vi "Motor with Encoder.vi"() -> ()   [LabVIEW 2016]
doc: "This example shows how to move a motor connected to an encoder and a wheel, and then read information about the system from an encoder.\n\nThis is an example of how to use feedback (from the encoder) to create an open loop system. If some control method was used, for example using PID, a closed loop system could be created.\n\nThis example expects a USB cable connected from your development PC to the Type B USB Jack (next to the power input) on the roboRIO.\n\nThis example requires the Driver Station to be running with Teleoperated Enabled."
uses:
  <vilib>/Rock Robotics/SystemInterfaces/DIO/FPGA_DIOChannel.ctl
  <vilib>/Rock Robotics/WPI/Encoder/WPI_EncoderType.ctl
  <vilib>/Rock Robotics/SystemInterfaces/DIO/FPGA_DIOPWMChannel.ctl
  <vilib>/Rock Robotics/WPI/Counter/WPI_CounterDigitalInputToDigitalSource.vi
  <vilib>/Rock Robotics/WPI/MotorControl/WPI_MotorControlOpen Talon.vi
panel:
  out "Current angle (deg)":dbl(knob) scale=0.0..360.0
  out "Distance (in)":dbl
  out "Revolutions":dbl
  in  "Wheel diameter (in)":dbl=6.0
  in  "Motor Speed (-1 to 1)":dbl(slide) scale=-1.0..1.0
  in  "Motor PWM Channel":T1
  in  "Number Samples to Average":u8=1 min=1 max=128
  in  "Invert Direction":bool
  in  "Decoding Type":T2=enum."4x"
  in  "DistancePerCount (deg)":dbl=0.288
  in  "Encoder B Channel":T3=enum."DIO 1"
  in  "Encoder A Channel":T3
  out "Encoder Rate (deg/sec)":dbl
  in  "Minimum Rate":dbl=20.0
  in  "Stop":bool
  in  "Reset Encoder?":bool
  out "Encoder Alarm Status":string
  out "Encoder Direction":string
  # "Set these inputs before running."
  # "These can be set while running."
  # "Output information."
  # "This example requires the Driver Station to be running with Teleoperated Enabled."
  # "PWM cable"
  # "This shows wiring for a Talon speed controller.  The wiring is similar for Victor and Jaguar controllers.  If you change the controller type, you must also select the appropriate instance of the Motor Open VI on the diagram."
  # "Power\nTerminals"
  # "Motor\nTerminals"
  # "+"
  # "+"
  # "M"
  # "B"
  # "Encoder\nB (white wire)---------\nGnd (black wire)------\n+5V (red wire)---------\nA (white wire)---------"
  # "roboRIO\nDIO-1  S\nDIO-0 \nDIO-0  V\nDIO-0  S"
  # "Encoder"
  # "Index"
  # "Gnd"
  # "+5V"
  # "B"
  # "A"
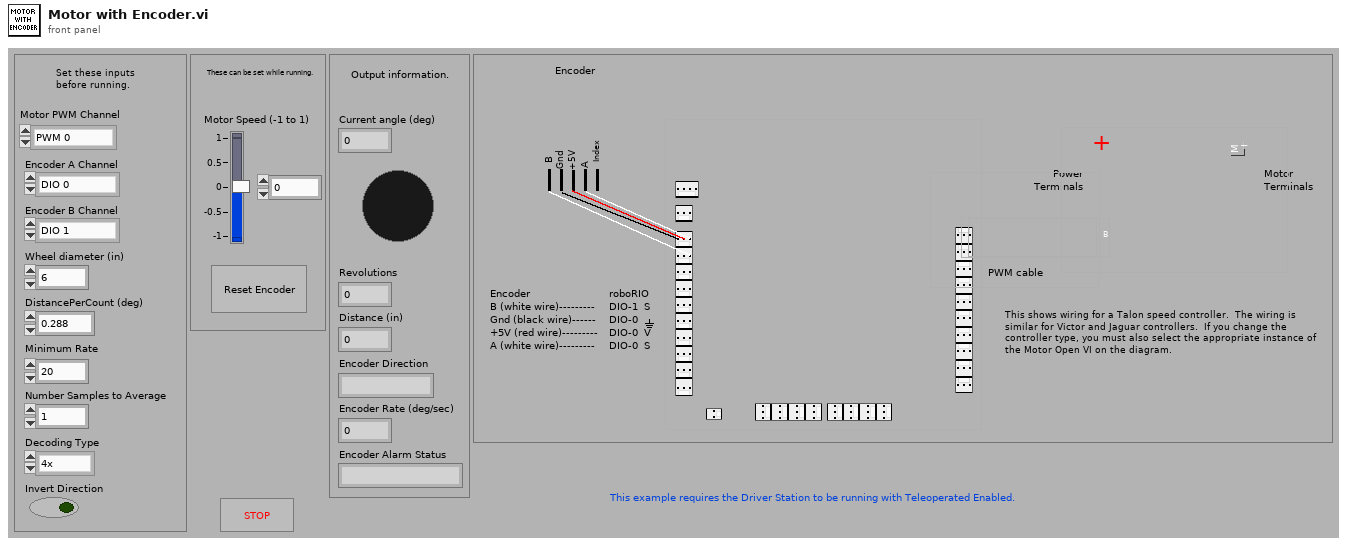
[diagram p1: front panel]
types:
  T1 = typedef "FPGA_DIOPWMChannel.ctl" = enum8{"PWM 0", "PWM 1", "PWM 2", "PWM 3", "PWM 4", "PWM 5", "PWM 6", "PWM 7", "PWM 8", "PWM 9", "PWM MXP 0", "PWM MXP 1", "PWM MXP 2", "PWM MXP 3", "PWM MXP 4", "PWM MXP 5", "PWM MXP 6", "PWM MXP 7", "PWM MXP 8", "PWM MXP 9", "Invalid"}
  T2 = typedef "WPI_EncoderType.ctl" = enum16{"1x", "2x", "4x"}
  T3 = typedef "FPGA_DIOChannel.ctl" = enum8{"DIO 0", "DIO 1", "DIO 2", "DIO 3", "DIO 4", "DIO 5", "DIO 6", "DIO 7", "DIO 8", "DIO 9", "DIO MXP 0", "DIO MXP 1", "DIO MXP 2", "DIO MXP 3", "DIO MXP 4", "DIO MXP 5", "DIO MXP 6", "DIO MXP 7", "DIO MXP 8", "DIO MXP 9", "DIO MXP 10", "DIO MXP 11", "DIO MXP 12", "DIO MXP 13", "DIO MXP 14", "DIO MXP 15", "SPI Port CS1", "SPI Port CS2", "SPI Port CS3", "SPI Port MISO", "SPI Port MOSI", "Invalid"}
  T4 = typedef "WPI_MotorControlDeviceRef.ctl" = cluster{"DeviceStatus":errorcluster, "Type":T5, "PWM":cluster{"PWM Channel":T1, "DeadBand":T6}, "CAN":cluster{"Device Number":u8, "SetOutput VI Ref":variant, "GetOutput VI Ref":variant, "Enable VI Ref":variant, "Disable VI Ref":variant, "Data":variant}, "Invert":bool}
  T5 = typedef "WPI_MotorControlType.ctl" = enum16{"PWM", "CAN"}
  T6 = typedef "WPI_PWMDeadband.ctl" = cluster{"Name":string, "maxPositivePwm":i32, "minPositivePwm":i32, "centerPwm":i32, "maxNegativePwm":i32, "minNegativePwm":i32, "angularRange":u16}
  T7 = typedef "WPI_DigitalInputDevRef.ctl" = cluster{"DevStatus":errorcluster, "DIO Channel":T3}
  T8 = typedef "FPGA_CounterEncoderSourceConvertionLVSourceType.ctl" = cluster{"DevStatus":errorcluster, "AnalogTriggerMode?":bool, "DigitalMode":cluster{"DIO Channel":T9}, "AnalogTriggerMode":cluster{"AnalogTriggerIndex":T10, "OutputType":T11}}
  T9 = typedef "FPGA_DIODigitalSourceChannel.ctl" = enum8{"DIO 0", "DIO 1", "DIO 2", "DIO 3", "DIO 4", "DIO 5", "DIO 6", "DIO 7", "DIO 8", "DIO 9", "DIO MXP 0", "DIO MXP 1", "DIO MXP 2", "DIO MXP 3", "DIO MXP 4", "DIO MXP 5", "DIO MXP 6", "DIO MXP 7", "DIO MXP 8", "DIO MXP 9", "DIO MXP 10", "DIO MXP 11", "DIO MXP 12", "DIO MXP 13", "DIO MXP 14", "DIO MXP 15", "Disabled"}
  T10 = typedef "FPGA_AnalogTriggerIndex.ctl" = enum8{"Trig 0", "Trig 1", "Trig 2", "Trig 3", "Trig 4", "Trig 5", "Trig 6", "Trig 7", "Invalid"}
  T11 = typedef "FPGA_AnalogTriggerOutType.ctl" = enum16{"InWindow", "TriggerState", "Rising", "Falling"}
  T12 = typedef "WPI_EncoderDevRef.ctl" = cluster{"DevStatus":errorcluster, "EncoderIndex":T13, "CounterIndex":T14, "DistancePerCount":dbl, "Decoding Type":T2}
  T13 = typedef "FPGA_EncoderIdx.ctl" = enum8{"Enc 0", "Enc 1", "Enc 2", "Enc 3", "Enc 4", "Enc 5", "Enc 6", "Enc 7", "Invalid"}
  T14 = typedef "FPGA_CounterCtrSystemIndex.ctl" = enum8{"Ctr 0", "Ctr 1", "Ctr 2", "Ctr 3", "Ctr 4", "Ctr 5", "Ctr 6", "Ctr 7", "Invalid"}
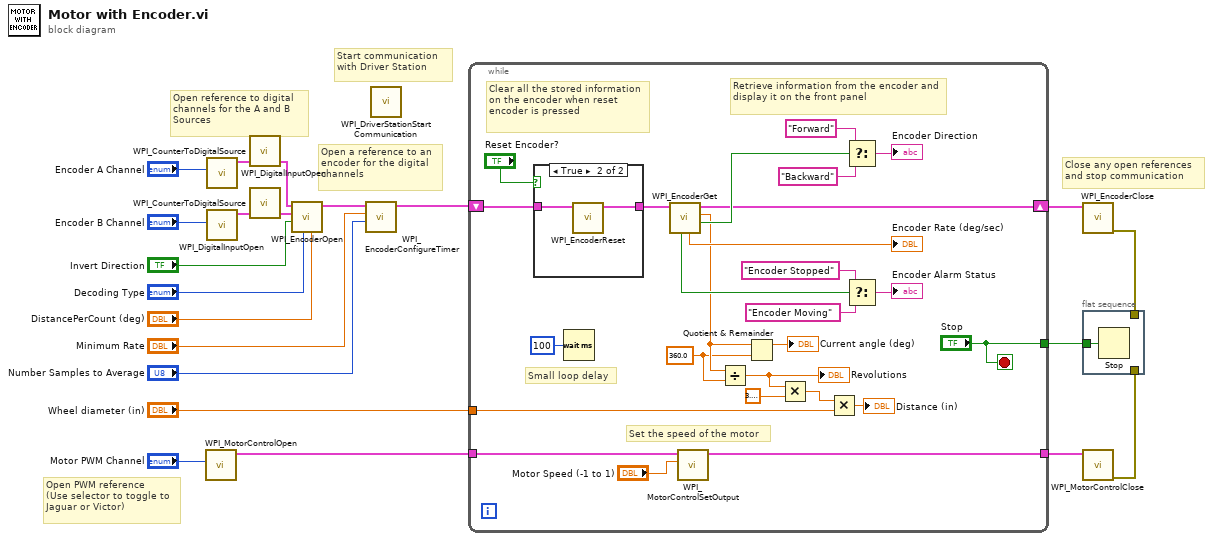
[diagram p0: block diagram]
diagram:
  # "Open PWM reference\n(Use selector to toggle to Jaguar or Victor)"
  # "Start communication with Driver Station"
  # "Close any open references\nand stop communication"
  # "Open a reference to an\nencoder for the digital \nchannels"
  # "Open reference to digital \nchannels for the A and B\nSources"
  n1 = call-poly <vilib>:"WPI_MotorControlOpen.vi"("PWM Channel"="Motor PWM Channel") -> ("MotorControlDeviceRef"=w5:T4)  [unwired: 3 in, 7 out]
  n2 = call <vilib>:"WPI_DigitalInputOpen.vi"("DIO Channel"="Encoder A Channel") -> ("DigitalInputDevRef"=w18:T7)  [unwired: 1 in, 9 out]
  n3 = call <vilib>:"WPI_DigitalInputOpen.vi"("DIO Channel"="Encoder B Channel") -> ("DigitalInputDevRef"=w19:T7)  [unwired: 1 in, 9 out]
  n4 = call-poly <vilib>:"WPI_CounterToDigitalSource.vi"("DigitalInputDevRef"=w18) -> ("Digital Source"=w17:T8)  [unwired: 6 out]
  n5 = call-poly <vilib>:"WPI_CounterToDigitalSource.vi"("DigitalInputDevRef"=w19) -> ("Digital Source"=w20:T8)  [unwired: 6 out]
  n6 = call <vilib>:"WPI_EncoderOpen.vi"("DistancePerCount"="DistancePerCount (deg)", "Decoding Type"="Decoding Type", "Invert Direction (False)"="Invert Direction", "BSource"=w20, "ASource"=w17) -> ("EncoderDevRef"=w10:T12)  [unwired: 3 in, 3 out]
  n7 = call <vilib>:"WPI_EncoderConfigureTimer.vi"("Number Samples to Average"="Number Samples to Average", "Minimum Rate"="Minimum Rate", "EncoderDevRef"=w10) -> ("EncoderDevRef"=w11:T12)  [unwired: 1 in, 7 out]
  n8 = call <vilib>:"WPI_DriverStationStart Communication.vi"() -> ()  [unwired: 2 in, 10 out]
  n9 = while {
    shift-right: [w40] -> w21
    shift-left: w11 -> [w45]
    tunnel: ["Stop"] -> w3
    tunnel: w5 -> [w33]
    tunnel: [w32] -> w7
    tunnel: "Wheel diameter (in)" -> [w27]
    stop <- "Stop" stop-if-true
    w30 = 360.0 ("y")
    # "Retrieve information from the encoder and display it on the front panel"
    # "Set the speed of the motor"
    # "Small loop delay"
    # "Clear all the stored information on the encoder when reset encoder is pressed"
    n10 = case shown="True" "Reset Encoder?" {
      tunnel: w45 -> [w48 w50]
      tunnel: [w48 w49] -> w43
      frame False {
      }
      frame True {
        n11 = call <vilib>:"WPI_EncoderReset.vi"("EncoderDevRef"=w50) -> ("EncoderDevRef"=w49:T12)  [unwired: 1 in, 9 out]
      }
    }
    n12 = Wait (ms)(milliseconds to wait=u32 100) -> ()  [unwired: 1 out]
    n13 = call <vilib>:"WPI_EncoderGet.vi"("EncoderDevRef"=w43) -> ("Direction"=w42:bool, "Distance"=w31:dbl, "EncoderDevRef"=w40:T12, "Rate"=→"Encoder Rate (deg/sec)":dbl, "Stopped"=w41:bool)  [unwired: 1 in, 5 out]
    n14 = call <vilib>:"WPI_MotorControlSetOutput.vi"("Output"="Motor Speed (-1 to 1)", "MotorControlDevRef"=w33) -> ("MotorControlDevRef"=w32:T4)  [unwired: 2 in, 7 out]
    n15 = Divide(x=w31, y=w30) -> (x/y=w29:dbl)
    "Revolutions" <- w29
    n16 = Quotient & Remainder(x=w31, y=w30) -> (x-y*floor(x/y)=→"Current angle (deg)":dbl)  [unwired: 1 out]
    n17 = Multiply(x=w29, y=3.141592653589793) -> (x*y=w25:dbl)
    n18 = Multiply(x=w25, y=w27) -> (x*y=→"Distance (in)":dbl)
    n19 = Select(t="Forward", s=w42, f="Backward") -> (s? t:f=→"Encoder Direction":string)
    n20 = Select(t="Encoder Stopped", s=w41, f="Encoder Moving") -> (s? t:f=→"Encoder Alarm Status":string)
  }
  n21 = call <vilib>:"WPI_EncoderClose.vi"("EncoderDevRef"=w21) -> ("error out"=w2:errorcluster)  [unwired: 2 in, 8 out]
  n22 = flat-sequence {
    tunnel: w3 -> [w51]
    tunnel: w2 -> [_]
    tunnel: w1 -> [_]
    frame #0 {
      n23 = Stop(stop? (T)=w51) -> ()
    }
  }
  n24 = call <vilib>:"WPI_MotorControlClose.vi"("MotorControlDevRef"=w7) -> ("error out"=w1:errorcluster)  [unwired: 1 in, 9 out]
